vi "Q3.vi"() -> ()   [LabVIEW 2020]
uses:
  54402a8a-6335-4590-be97-694ebf0c10c0.vi
  <vilib>/Array/Sort 2D Array - Pop Stack.vi
  <vilib>/Array/Sort 2D Array - Push Stack.vi
  54402a8a-6335-4590-be97-694ebf0c10c0.vi/269d4b3b-47f5-49e3-8884-44851e4dd9d5.vi
  54402a8a-6335-4590-be97-694ebf0c10c0.vi/6d99389c-673d-4efb-bf33-19b32bcf4cf8.vi
  <vilib>/Utility/file.llb/Read Delimited Spreadsheet (DBL).vi
panel:
  out "Slope":dbl
  out "Intercept":dbl
  out "3c":cluster{dbl[], dbl[]}[](graph)
  out "3b":dbl[][](array[numeric])
  out "3a":dbl[][](array[numeric])
  out "3a":cluster{"Y":dbl[], "Y":dbl[]}[](graph)
  in  "file path (dialog if empty)":path
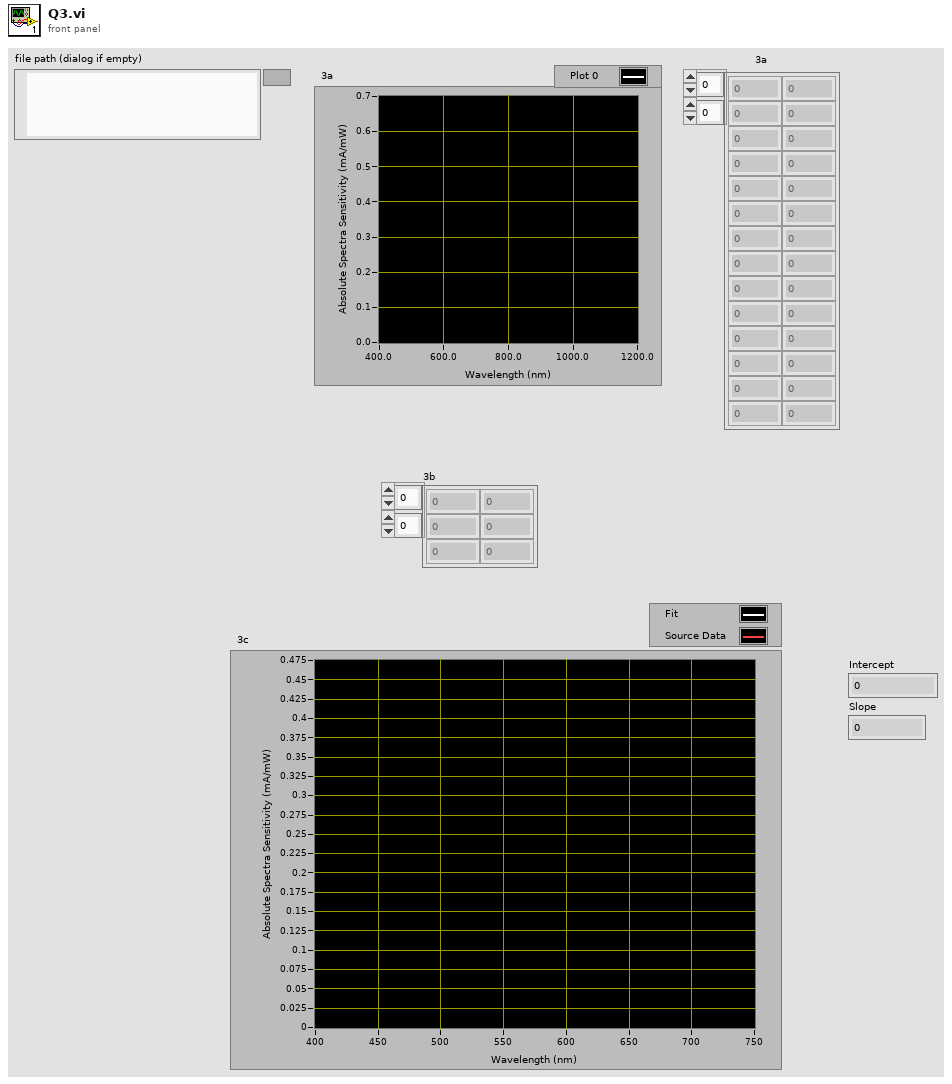
[diagram p1: front panel]
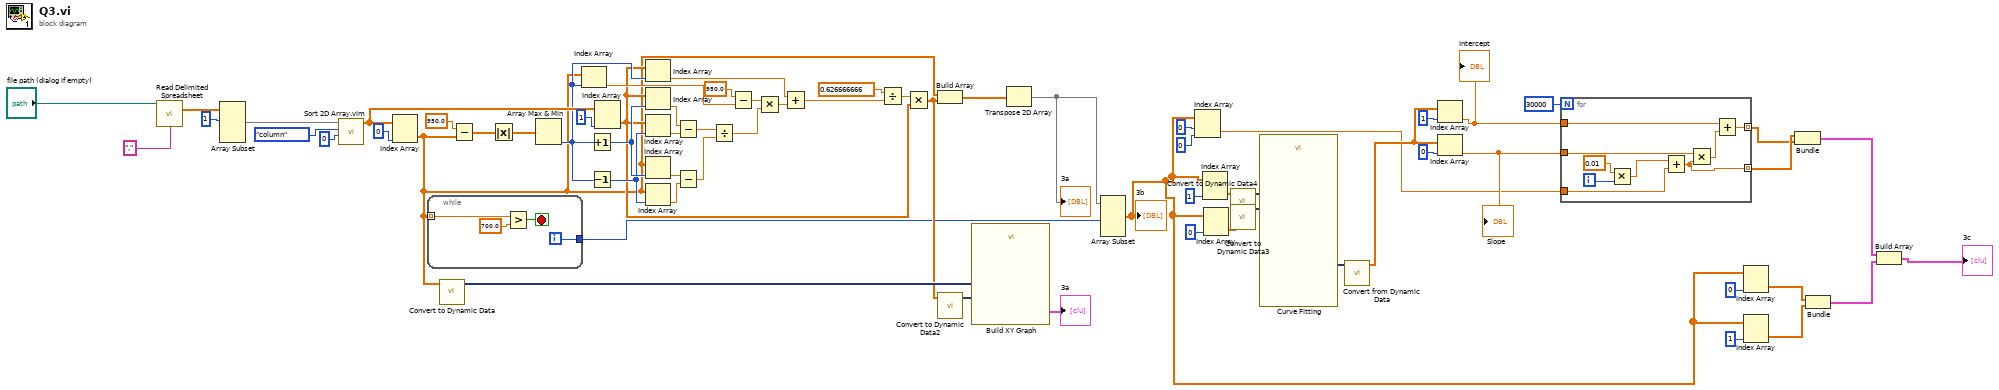
[diagram p0: block diagram]
diagram:
  n1 = call-poly <vilib>:"Read Delimited Spreadsheet.vi"("file path (dialog if empty)"="file path (dialog if empty)", "delimiter (\\t)"="," ("delimiter (\\t)")) -> ("all rows"=w63:dbl[][])  [unwired: 8 in, 5 out]
  n2 = Array Subset(array=w63, index (row)=1 ("index")) -> (w30:dbl[][])  [unwired: 3 in]
  n3 = call "Sort 2D Array.vim"("index"=0, "dimension to index (column)"=enum16{"column", "row"}."column", "2D array"=w30) -> ("sorted 2D array"=w58:dbl[][])  [unwired: 7 in, 1 out]
  n4 = Index Array(array=w58, index (col)=0 ("disabled index (col)")) -> (element=w29:dbl[])  [unwired: 1 in]
  n5 = while {
    tunnel: w29 -> [w68] mode=indexing
    tunnel: [w67] -> w27
    i -> [w67]
    stop <- w69 stop-if-true
    n6 = Greater?(x=w68, y=700.0) -> (0:w69:bool)
  }
  n7 = call "Convert to Dynamic Data"("Array"=w29) -> ("Dynamic Data Type"=w59:dynamicdata)  [unwired: 3 in]
  n8 = Subtract(x=950.0 ("y"), y=w29) -> (x-y=w54:dbl[])
  n9 = Absolute Value(x=w54) -> (abs(x)=w53:dbl[])
  n10 = Array Max & Min(array=w53) -> (min index (indices)=w45:i32)  [unwired: 3 out]
  n11 = Index Array(array=w29, index=w45) -> (element=w40:dbl)
  n12 = Increment(x=w45) -> (x+1=w52:i32)
  n13 = Decrement(x=w45) -> (x-1=w51:i32)
  n14 = Index Array(array=w58, index (col)=1 ("disabled index (col)")) -> (element=w36:dbl[])  [unwired: 1 in]
  n15 = Index Array(array=w36, index=w45) -> (element=w46:dbl)
  n16 = Index Array(array=w36, index=w52) -> (element=w48:dbl)
  n17 = Index Array(array=w36, index=w51) -> (element=w47:dbl)
  n18 = Index Array(array=w29, index=w52) -> (element=w50:dbl)
  n19 = Index Array(array=w29, index=w51) -> (element=w49:dbl)
  n20 = Subtract(x=w48, y=w47) -> (x-y=w33:dbl)
  n21 = Subtract(x=w50, y=w49) -> (x-y=w34:dbl)
  n22 = Divide(x=w33, y=w34) -> (x/y=w43:dbl)
  n23 = Subtract(x=950.0 ("y"), y=w40) -> (x-y=w44:dbl)
  n24 = Multiply(x=w44, y=w43) -> (x*y=w42:dbl)
  n25 = Add(x=w46, y=w42) -> (x+y=w39:dbl)
  n26 = Divide(x=0.626666666, y=w39) -> (x/y=w37:dbl)
  n27 = Multiply(x=w37, y=w36) -> (x*y=w32:dbl[])
  n28 = Build Array(w29, w32) -> (w31:dbl[][])
  n29 = call "Convert to Dynamic Data2"("Array"=w32) -> ("Dynamic Data Type"=w35:dynamicdata)  [unwired: 3 in]
  n30 = call "Build XY Graph"("Y Input"=w35, "X Input"=w59) -> ("XY Graph"=→"3a":cluster{"X":dbl[], "Y":dbl[]}[])  [unwired: 8 in, 1 out]
  n31 = Transpose 2D Array(2D array=w31) -> (transposed array=w28:dbl[][])
  "3a" <- w28
  n32 = Array Subset(array=w28, length (row)=w27) -> (w10:dbl[][])  [unwired: 3 in]
  "3b" <- w10
  n33 = Index Array(array=w10, index (row)=0, index (col)=0 ("disabled index (col)")) -> (element=w3:dbl)
  n34 = Index Array(array=w10, index (col)=1 ("disabled index (col)")) -> (element=w7:dbl[])  [unwired: 1 in]
  n35 = Index Array(array=w10, index (col)=0 ("disabled index (col)")) -> (element=w9:dbl[])  [unwired: 1 in]
  n36 = call "Convert to Dynamic Data4"("Array"=w7) -> ("Dynamic Data Type"=w6:dynamicdata)  [unwired: 3 in]
  n37 = call "Convert to Dynamic Data3"("Array"=w9) -> ("Dynamic Data Type"=w8:dynamicdata)  [unwired: 3 in]
  n38 = call "Curve Fitting"("Locations"=w8, "Signals"=w6) -> ("general LS coefficients"=w26:dynamicdata)  [unwired: 5 in, 4 out]
  n39 = call "Convert from Dynamic Data"("Dynamic Data Type"=w26) -> ("Array"=w25:dbl[])  [unwired: 3 in]
  n40 = Index Array(array=w25, index=1) -> (element=w2:dbl)
  "Intercept" <- w2
  n41 = Index Array(array=w25, index=0) -> (element=w20:dbl)
  "Slope" <- w20
  n42 = for {
    N: 30000 -> [_]
    tunnel: w20 -> [w79]
    tunnel: [w75] -> w18 mode=indexing
    tunnel: [w73] -> w19 mode=indexing
    tunnel: w3 -> [w72]
    tunnel: w2 -> [w71]
    i -> [w78]
    n43 = Multiply(x=0.01, y=w78) -> (x*y=w74:dbl)
    n44 = Add(x=w74, y=w72) -> (x+y=w73:dbl)
    n45 = Multiply(x=w79, y=w73) -> (x*y=w76:dbl)
    n46 = Add(x=w71, y=w76) -> (x+y=w75:dbl)
  }
  n47 = Index Array(array=w10, index (col)=0 ("disabled index (col)")) -> (element=w15:dbl[])  [unwired: 1 in]
  n48 = Index Array(array=w10, index (col)=1 ("disabled index (col)")) -> (element=w14:dbl[])  [unwired: 1 in]
  n49 = Bundle(w19, w18) -> (w12:cluster{dbl[], dbl[]})  [unwired: 1 in]
  n50 = Bundle(w15, w14) -> (w13:cluster{dbl[], dbl[]})  [unwired: 1 in]
  n51 = Build Array(w12, w13) -> (→"3c":cluster{dbl[], dbl[]}[])
